vi "Register Project View.vi"(11 "Message Enqueuer in":refnum<class "Message Enqueuer.lvclass">) -> (3 "Message Enqueuer out":refnum<class "Message Enqueuer.lvclass">)   [LabVIEW 2013]
uses:
  <vilib>/ActorFramework/Message Enqueuer/Message Enqueuer.lvclass
  <vilib>/ActorFrameworkMVC/View Observer/Registration Message/Registration Message.lvclass
  <vilib>/ActorFrameworkMVC/View Observer/Data Message/Data Message.lvclass
  Models/Project Model Messages/Register Tiles Info Msg/Register Tiles Info Msg.lvclass
  Models/Project Model Messages/Register Previous Button Visibility Msg/Register Previous Button Visibility Msg.lvclass
  Models/Project Model Messages/Register Next Button Visibility Msg/Register Next Button Visibility Msg.lvclass
  Views/Project View Messages/Tiles Info Msg/Tiles Info Msg.lvclass
  Views/Project View Messages/Previous Button Visibility Msg/Previous Button Visibility Msg.lvclass
  Views/Project View Messages/Next Button Visibility Msg/Next Button Visibility Msg.lvclass
  Models/Project Model Messages/Register Move In Previous Msg/Register Move In Previous Msg.lvclass
  Views/Project View Messages/Conceret Move In Previous Msg/Conceret Move In Previous Msg.lvclass
  Models/Project Model Messages/Register Move In Next Msg/Register Move In Next Msg.lvclass
  Views/Project View Messages/Conceret Move In Next Msg/Conceret Move In Next Msg.lvclass
  <vilib>/ActorFrameworkMVC/UI Controller Messages/Subscribe View to Model Msg/Subscribe View to Model Msg.lvclass/Subscribe View to Model Msg.ctl
  <vilib>/ActorFramework/Message Enqueuer/Message Enqueuer.lvclass/Message Enqueuer.ctl
  <vilib>/ActorFramework/Message Enqueuer/Enqueue.vi
  <vilib>/ActorFramework/Message Priority Queue/Priority Enqueue.vi
  <vilib>/ActorFrameworkMVC/UI Controller Messages/Subscribe View to Model Msg/Subscribe View to Model Msg.lvclass
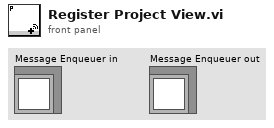
[diagram p1: front panel]
types:
  T1 = cluster{"Registration Message":string, "Data Message":string}[]
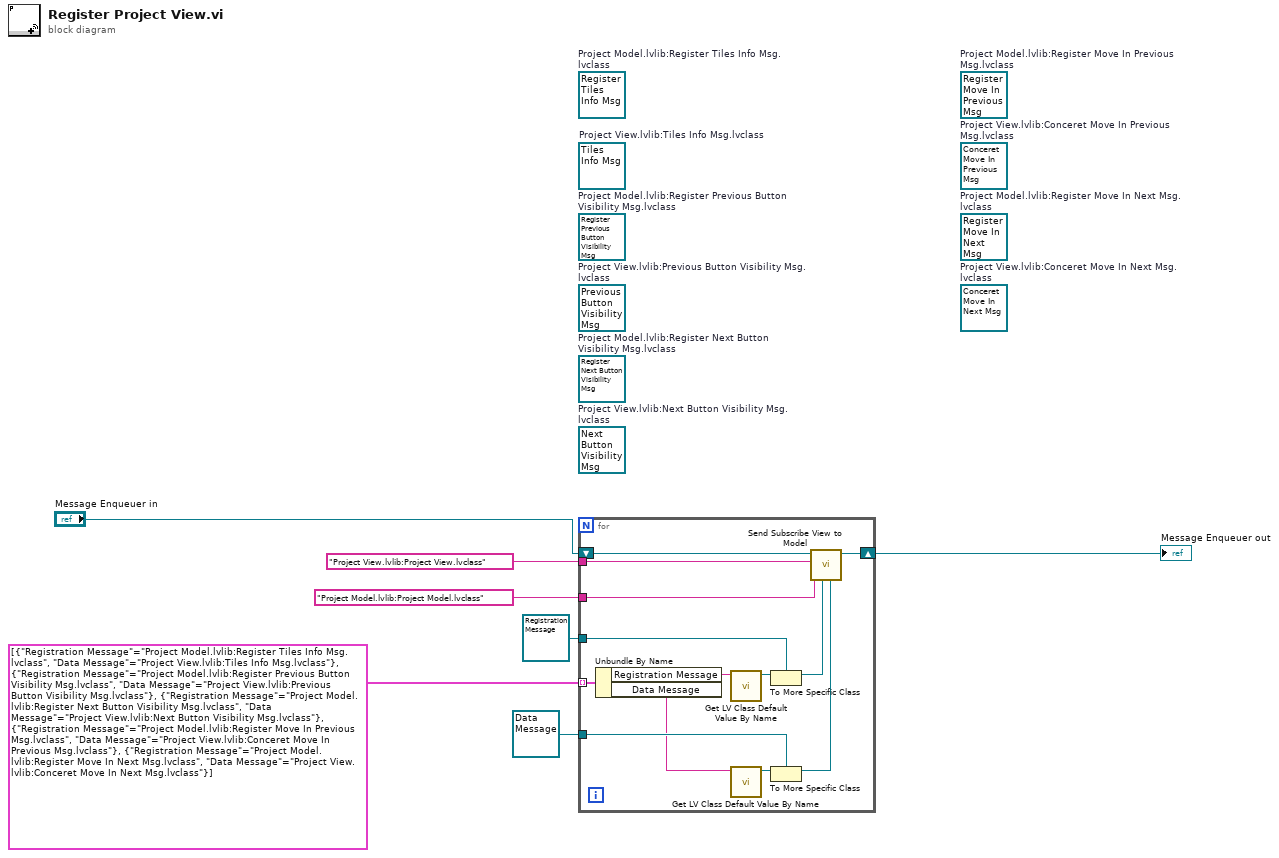
[diagram p0: block diagram]
diagram:
  (unwired) refnum<class "Conceret Move In Next Msg.lvclass"> refnum  # Project View.lvlib:Conceret Move In Next Msg.lvclass
  (unwired) refnum<class "Register Move In Next Msg.lvclass"> refnum  # Project Model.lvlib:Register Move In Next Msg.lvclass
  (unwired) refnum<class "Conceret Move In Previous Msg.lvclass"> refnum  # Project View.lvlib:Conceret Move In Previous Msg.lvclass
  (unwired) refnum<class "Register Move In Previous Msg.lvclass"> refnum  # Project Model.lvlib:Register Move In Previous Msg.lvclass
  (unwired) refnum<class "Next Button Visibility Msg.lvclass"> refnum  # Project View.lvlib:Next Button Visibility Msg.lvclass
  (unwired) refnum<class "Previous Button Visibility Msg.lvclass"> refnum  # Project View.lvlib:Previous Button Visibility Msg.lvclass
  (unwired) refnum<class "Tiles Info Msg.lvclass"> refnum  # Project View.lvlib:Tiles Info Msg.lvclass
  (unwired) refnum<class "Register Next Button Visibility Msg.lvclass"> refnum  # Project Model.lvlib:Register Next Button Visibility Msg.lvclass
  (unwired) refnum<class "Register Previous Button Visibility Msg.lvclass"> refnum  # Project Model.lvlib:Register Previous Button Visibility Msg.lvclass
  (unwired) refnum<class "Register Tiles Info Msg.lvclass"> refnum  # Project Model.lvlib:Register Tiles Info Msg.lvclass
  n1 = for {
    tunnel: "Project View.lvlib:Project View.lvclass" ("View Name") -> [w19]
    tunnel: "Project Model.lvlib:Project Model.lvclass" ("Model Name") -> [w18]
    shift-right: [w17] -> w7
    shift-left: "Message Enqueuer in" -> [w20]
    tunnel: refnum<class "Registration Message.lvclass"> refnum ("Registration Message") -> [w14]
    tunnel: refnum<class "Data Message.lvclass"> refnum ("Data Message") -> [w13]
    tunnel: T1 [{"Registration Message"="Project Model.lvlib:Register Tiles Info Msg.lvclass", "Data Message"="Project View.lvlib:Tiles Info Msg.lvclass"}, {"Registration Message"="Project Model.lvlib:Register Previous Button Visibility Msg.lvclass", "Data Message"="Project View.lvlib:Previous Button Visibility Msg.lvclass"}, {"Registration Message"="Project Model.lvlib:Register Next Button Visibility Msg.lvclass", "Data Message"="Project View.lvlib:Next Button Visibility Msg.lvclass"}, {"Registration Message"="Project Model.lvlib:Register Move In Previous Msg.lvclass", "Data Message"="Project View.lvlib:Conceret Move In Previous Msg.lvclass"}, {"Registration Message"="Project Model.lvlib:Register Move In Next Msg.lvclass", "Data Message"="Project View.lvlib:Conceret Move In Next Msg.lvclass"}] -> [w12] mode=indexing
    n2 = Unbundle By Name(w12) -> ("Registration Message"=w9:string, "Data Message"=w8:string)
    n3 = call <vilib>:"Get LV Class Default Value By Name.vi"("class name"=w9) -> ("object"=w16:refnum<class>)  [unwired: 9 in, 1 out]
    n4 = call <vilib>:"Get LV Class Default Value By Name.vi"("class name"=w8) -> ("object"=w15:refnum<class>)  [unwired: 9 in, 1 out]
    n5 = To More Specific Class(target class=w14, reference=w16) -> (specific class reference=w11:refnum<class "Registration Message.lvclass">)  [unwired: 1 in, 1 out]
    n6 = To More Specific Class(target class=w13, reference=w15) -> (specific class reference=w10:refnum<class "Data Message.lvclass">)  [unwired: 1 in, 1 out]
    n7 = call <vilib>:"Send Subscribe View to Model.vi"("Data Message"=w10, "Registration Message"=w11, "Model Name"=w18, "View Name"=w19, "Message Enqueuer"=w20) -> ("Message Enqueuer out"=w17:refnum<class "Message Enqueuer.lvclass">)  [unwired: 5 in, 1 out]
  }
  "Message Enqueuer out" <- w7
